vi "KE22XX_Basic_All_CH_Setting.vi"(0 "VISA In":refnum<visa-resource-name>, 1 "Channe 1":T1, 2 "Channe 2":T1, 3 "Channe 3":T1, 5 "ID ?":bool, 7 "Remote":bool, 9 "Reset":bool, 11 "error in":errorcluster) -> (15 "error out":errorcluster)   [LabVIEW 2016]
uses:
  Channel Control.ctl
  <userlib>/_TI-LA/Instr Drivers/Power Supply/KE22xx/Driver/Base/Keithley KE22xx Series.lvlib
panel:
  in  "Tab Control":enum32{"Channel 1", "Channel 2", "Channel 3"}(tab)
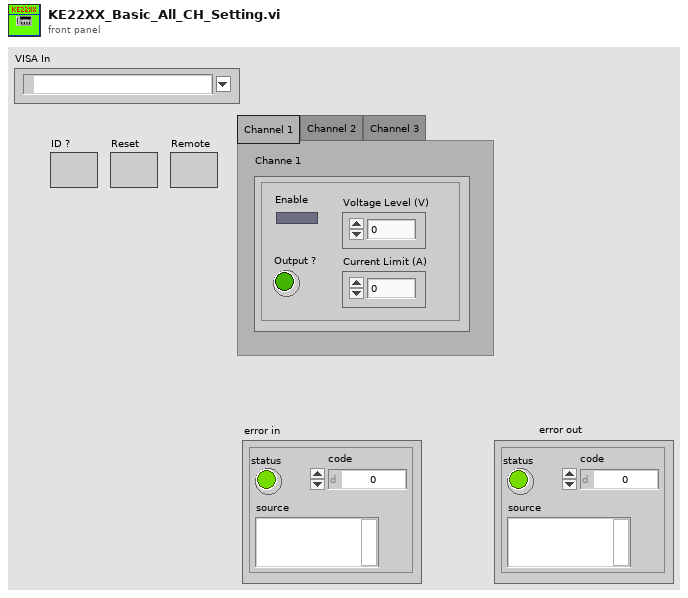
[diagram p1: front panel]
types:
  T1 = typedef "Channel Control.ctl" = cluster{"Output ?":bool, "Enable":bool, "Voltage Level (V)":dbl, "Current Limit (A) ":dbl}
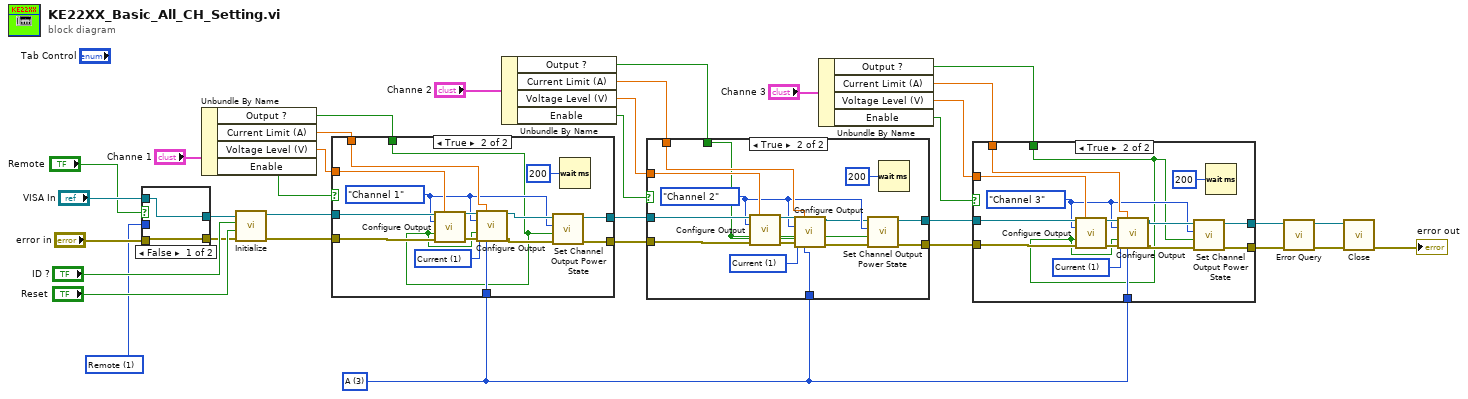
[diagram p0: block diagram]
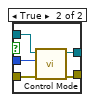
[diagram p2: hidden frame]
diagram:
  w2 = u16 3 items=["V", "mV", "kV", "A", "mA"] ("Unit(V)")
  w3 = u16 1 items=["Local", "Remote", "Remote Lock"] ("Control Mode (1: Remote)")
  n1 = case shown="False" "Remote" {
    tunnel: [w37 w42] -> w7
    tunnel: "VISA In" -> [w37 w41]
    tunnel: "error in" -> [w36 w40]
    tunnel: [w36 w39] -> w4
    tunnel: w3 -> [_ w38]
    frame False {
    }
    frame True {
      n2 = call <userlib>:"Control Mode.vi"("error in (no error)"=w40, "Control Mode (1: Remote)"=w38, "VISA resource name"=w41) -> ("error out"=w39:errorcluster, "VISA resource name out"=w42:refnum<visa-resource-name>)  [unwired: 7 in]
    }
  }
  n3 = Unbundle By Name("Channe 1") -> ("Output ?"=w27:bool, "Current Limit (A)"=w28:dbl, "Voltage Level (V)"=w29:dbl, "Enable"=w30:bool)
  n4 = call <userlib>:"Initialize.vi"("error in (no error)"=w4, "Reset (True)"="Reset", "ID Query (True)"="ID ?", "VISA resource name"=w7) -> ("error out"=w32:errorcluster, "VISA resource name out"=w33:refnum<visa-resource-name>)  [unwired: 6 in]
  n5 = case shown="True" w30 {
    tunnel: w33 -> [w43 w59]
    tunnel: w32 -> [w44 w58]
    tunnel: w29 -> [_ w57]
    tunnel: w28 -> [_ w49]
    tunnel: w27 -> [_ w46]
    tunnel: [w43 w56] -> w19
    tunnel: [w44 w55] -> w18
    tunnel: w2 -> [_ w48]
    frame False {
    }
    frame True {
      w52 = u16 1 items=["Voltage", "Current"] ("Function(0:Voltage)")
      w47 = enum16{"Channel 1", "Channel 2", "Channel 3"}."Channel 1" ("Channel Select")
      n6 = call <userlib>:"Configure Output.vi"("VISA resource name"=w59, "Manual Range(0.00)"=w57, "Channel Select"=w47, "Enable Output (T: Enable)"=w46, "error in (no error)"=w58) -> ("VISA resource name out"=w54:refnum<visa-resource-name>, "error out"=w53:errorcluster)  [unwired: 9 in]
      n7 = call <userlib>:"Configure Output.vi"("VISA resource name"=w54, "Manual Range(0.00)"=w49, "Channel Select"=w47, "Function(0:Voltage)"=w52, "Enable Output (T: Enable)"=w46, "error in (no error)"=w53, "Unit(V)"=w48) -> ("VISA resource name out"=w50:refnum<visa-resource-name>, "error out"=w51:errorcluster)  [unwired: 7 in]
      n8 = call <userlib>:"Set Channel Output Power State.vi"("error in (no error)"=w51, "Enable Output (T: On)"=w46, "Channel Select"=w47, "Visa Resource Name IN"=w50) -> ("error out"=w55:errorcluster, "Visa Resource Name OUT"=w56:refnum<visa-resource-name>)  [unwired: 6 in]
      n9 = Wait (ms)(milliseconds to wait=u32 200) -> ()  [unwired: 1 out]
    }
  }
  n10 = Unbundle By Name("Channe 2") -> ("Output ?"=w20:bool, "Current Limit (A)"=w21:dbl, "Voltage Level (V)"=w22:dbl, "Enable"=w23:bool)
  n11 = case shown="True" w23 {
    tunnel: w19 -> [w61 w76]
    tunnel: w18 -> [w60 w75]
    tunnel: w22 -> [_ w74]
    tunnel: w21 -> [_ w69]
    tunnel: w20 -> [_ w63]
    tunnel: [w61 w73] -> w12
    tunnel: [w60 w72] -> w11
    tunnel: w2 -> [_ w64]
    frame False {
    }
    frame True {
      w68 = u16 1 items=["Voltage", "Current"] ("Function(0:Voltage)")
      w67 = enum16{"Channel 1", "Channel 2", "Channel 3"}."Channel 2" ("Channel Select")
      n12 = call <userlib>:"Configure Output.vi"("VISA resource name"=w76, "Manual Range(0.00)"=w74, "Channel Select"=w67, "Enable Output (T: Enable)"=w63, "error in (no error)"=w75) -> ("VISA resource name out"=w71:refnum<visa-resource-name>, "error out"=w70:errorcluster)  [unwired: 9 in]
      n13 = call <userlib>:"Configure Output.vi"("VISA resource name"=w71, "Manual Range(0.00)"=w69, "Channel Select"=w67, "Function(0:Voltage)"=w68, "Enable Output (T: Enable)"=w63, "error in (no error)"=w70, "Unit(V)"=w64) -> ("VISA resource name out"=w65:refnum<visa-resource-name>, "error out"=w66:errorcluster)  [unwired: 7 in]
      n14 = call <userlib>:"Set Channel Output Power State.vi"("error in (no error)"=w66, "Enable Output (T: On)"=w63, "Channel Select"=w67, "Visa Resource Name IN"=w65) -> ("error out"=w72:errorcluster, "Visa Resource Name OUT"=w73:refnum<visa-resource-name>)  [unwired: 6 in]
      n15 = Wait (ms)(milliseconds to wait=u32 200) -> ()  [unwired: 1 out]
    }
  }
  n16 = Unbundle By Name("Channe 3") -> ("Output ?"=w13:bool, "Current Limit (A)"=w14:dbl, "Voltage Level (V)"=w15:dbl, "Enable"=w16:bool)
  n17 = case shown="True" w16 {
    tunnel: w12 -> [w78 w93]
    tunnel: w11 -> [w77 w92]
    tunnel: w15 -> [_ w91]
    tunnel: w14 -> [_ w85]
    tunnel: w13 -> [_ w80]
    tunnel: [w78 w90] -> w10
    tunnel: [w77 w89] -> w9
    tunnel: w2 -> [_ w82]
    frame False {
    }
    frame True {
      w86 = u16 1 items=["Voltage", "Current"] ("Function(0:Voltage)")
      w81 = enum16{"Channel 1", "Channel 2", "Channel 3"}."Channel 3" ("Channel Select")
      n18 = call <userlib>:"Configure Output.vi"("VISA resource name"=w93, "Manual Range(0.00)"=w91, "Channel Select"=w81, "Enable Output (T: Enable)"=w80, "error in (no error)"=w92) -> ("VISA resource name out"=w88:refnum<visa-resource-name>, "error out"=w87:errorcluster)  [unwired: 9 in]
      n19 = call <userlib>:"Configure Output.vi"("VISA resource name"=w88, "Manual Range(0.00)"=w85, "Channel Select"=w81, "Function(0:Voltage)"=w86, "Enable Output (T: Enable)"=w80, "error in (no error)"=w87, "Unit(V)"=w82) -> ("VISA resource name out"=w84:refnum<visa-resource-name>, "error out"=w83:errorcluster)  [unwired: 7 in]
      n20 = call <userlib>:"Set Channel Output Power State.vi"("error in (no error)"=w83, "Enable Output (T: On)"=w80, "Channel Select"=w81, "Visa Resource Name IN"=w84) -> ("error out"=w89:errorcluster, "Visa Resource Name OUT"=w90:refnum<visa-resource-name>)  [unwired: 6 in]
      n21 = Wait (ms)(milliseconds to wait=u32 200) -> ()  [unwired: 1 out]
    }
  }
  n22 = call <userlib>:"Error Query.vi"("error in (no error)"=w9, "VISA resource name"=w10) -> ("error out"=w26:errorcluster, "VISA resource name out"=w25:refnum<visa-resource-name>)  [unwired: 6 in, 2 out]
  n23 = call <userlib>:"Close.vi"("error in (no error)"=w26, "VISA resource name"=w25) -> ("error out"=→"error out":errorcluster)  [unwired: 9 in]
